vi "maxp.vi"() -> ()   [LabVIEW 2020]
uses:
  <vilib>/userdefined/High Color/IMAQdx.ctl
  C:/Users/lenovo/source/repos/MSMQ_try/how/bin/Release/how.dll
  source/repos/MSMQ_try/how/bin/Release/how.dll
  C:/Users/lenovo/source/repos/MSMQ_try/MIrror_x64/bin/Debug/MIrror_x64.dll
  source/repos/MSMQ_try/MIrror_x64/bin/Debug/MIrror_x64.dll
  <vilib>/vision/driver/NI_Vision_Acquisition_Software.lvlib
  source/repos/cont2019/x64/Release/Image_processing.dll
  <resource>/objmgr/imaqdx.rc
panel:
  in  "treshold":dbl=20000000.0
  out "st":bool
  out "ind":i32
  in  "ENA":bool
  in  "Relax":bool
  out "Power 2":dbl(graph)
  out "Power_val":dbl
  in  "stop 2":bool
  out "Image":T1(plugin-control)
  in  "Exposure time":dbl=1000.0
  out "FPS":dbl
  out "maximum":u8
  out "Power":dbl(graph)
  in  "Num frames":i32=3
  in  "Session In":T2="cam2"
  in  "amplitude_limit":dbl=0.1
  in  "phi_v":dbl
  in  "phi_g":dbl=1.6
  in  "phi_p":dbl=1.2
  in  "vel_limit":dbl=0.4
  in  "init_zero":bool
  out "Waveform Graph 2":dbl[](graph)
  in  "stop":bool
  out "mirror params":string
  in  "DM":bool
  out "Iterations":i32
  out "global_best_value":dbl
  out "Waveform Graph":dbl[](graph)
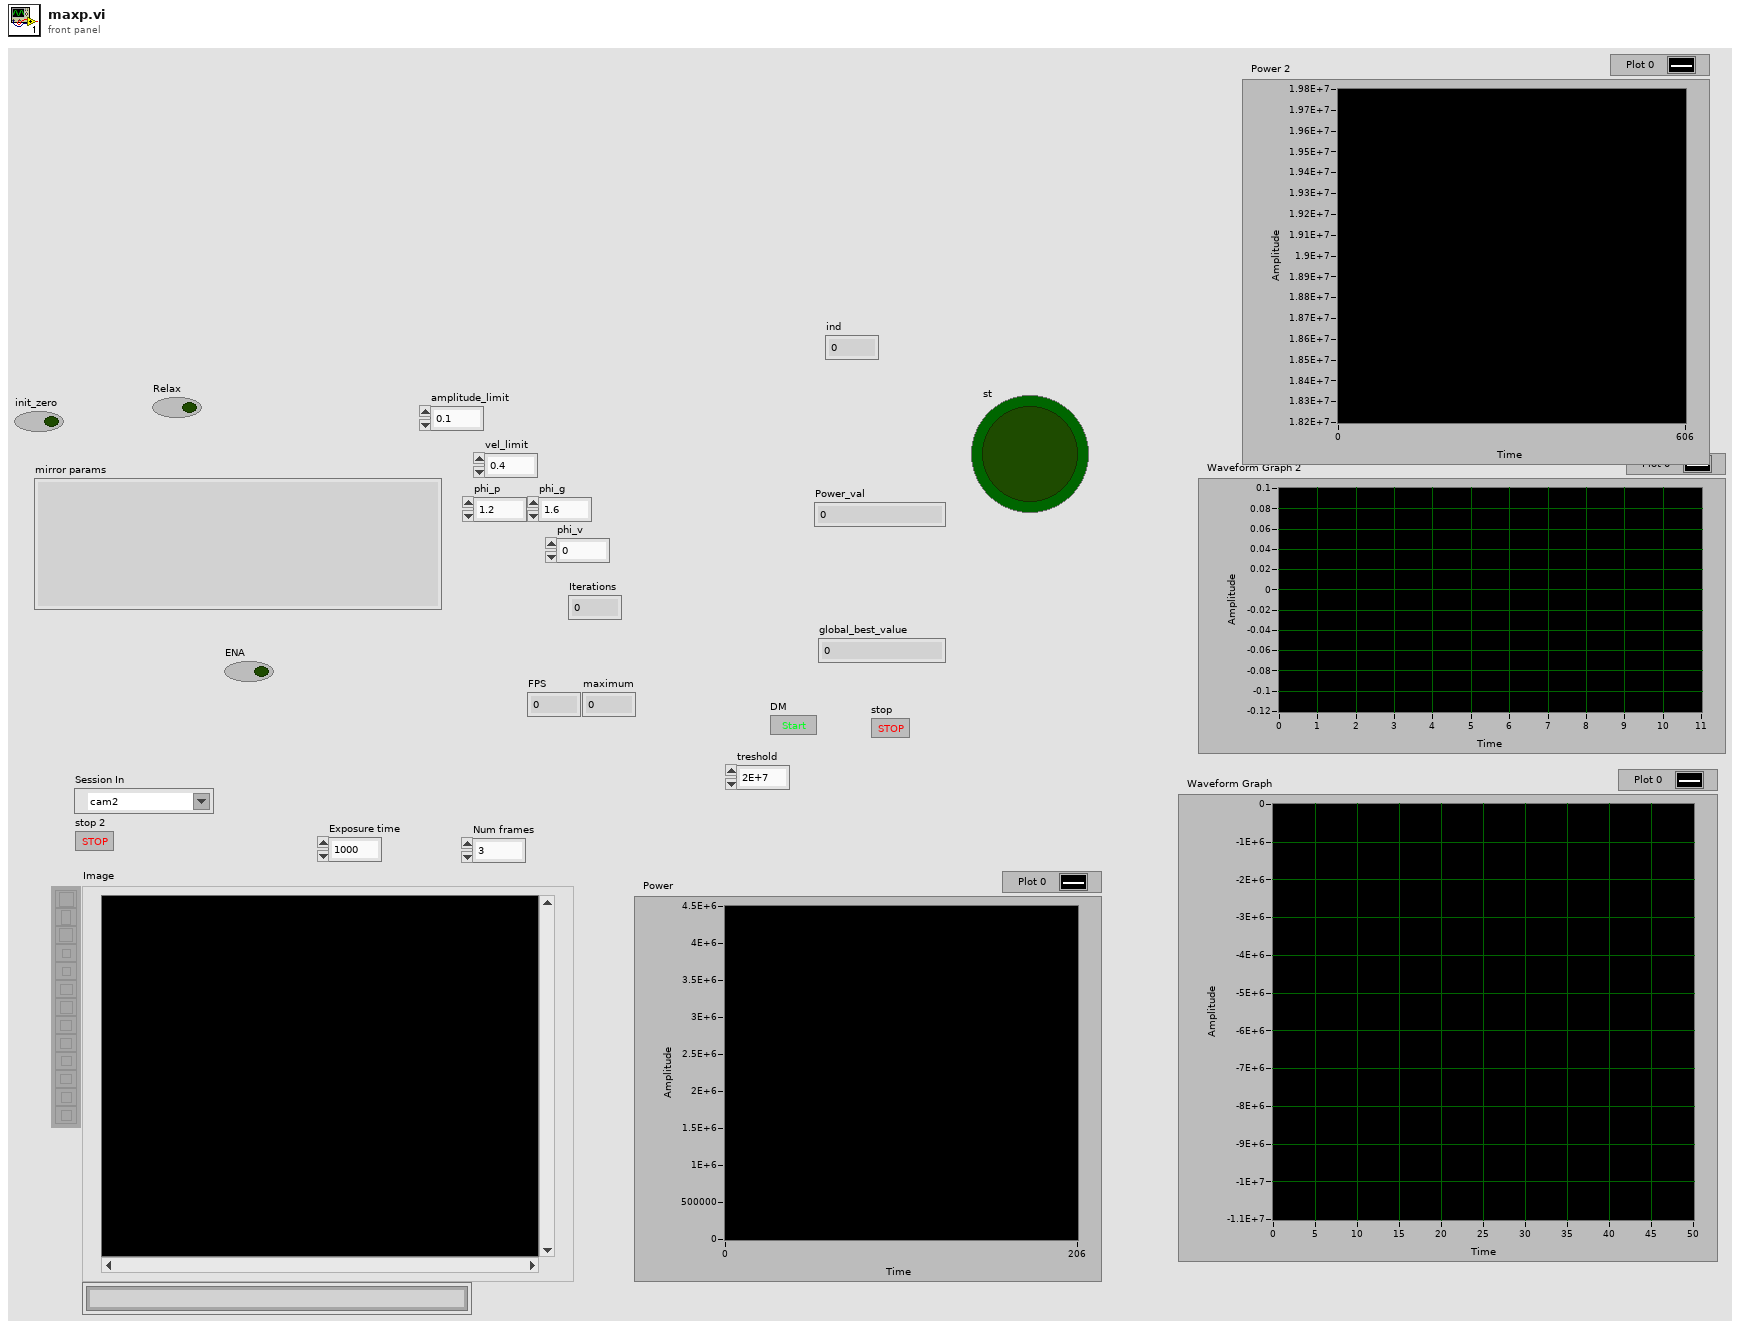
[diagram p1: front panel]
types:
  T1 = typedef "IMAQ Image.ctl" = refnum<image>
  T2 = typedef "IMAQdx.ctl" = refnum<k21>
  T3 = cluster{"Global Rectangle":i32[], "Contours":cluster{"Contour Type":u32, "ROI Type":u32, "Points":i32[]}[]}
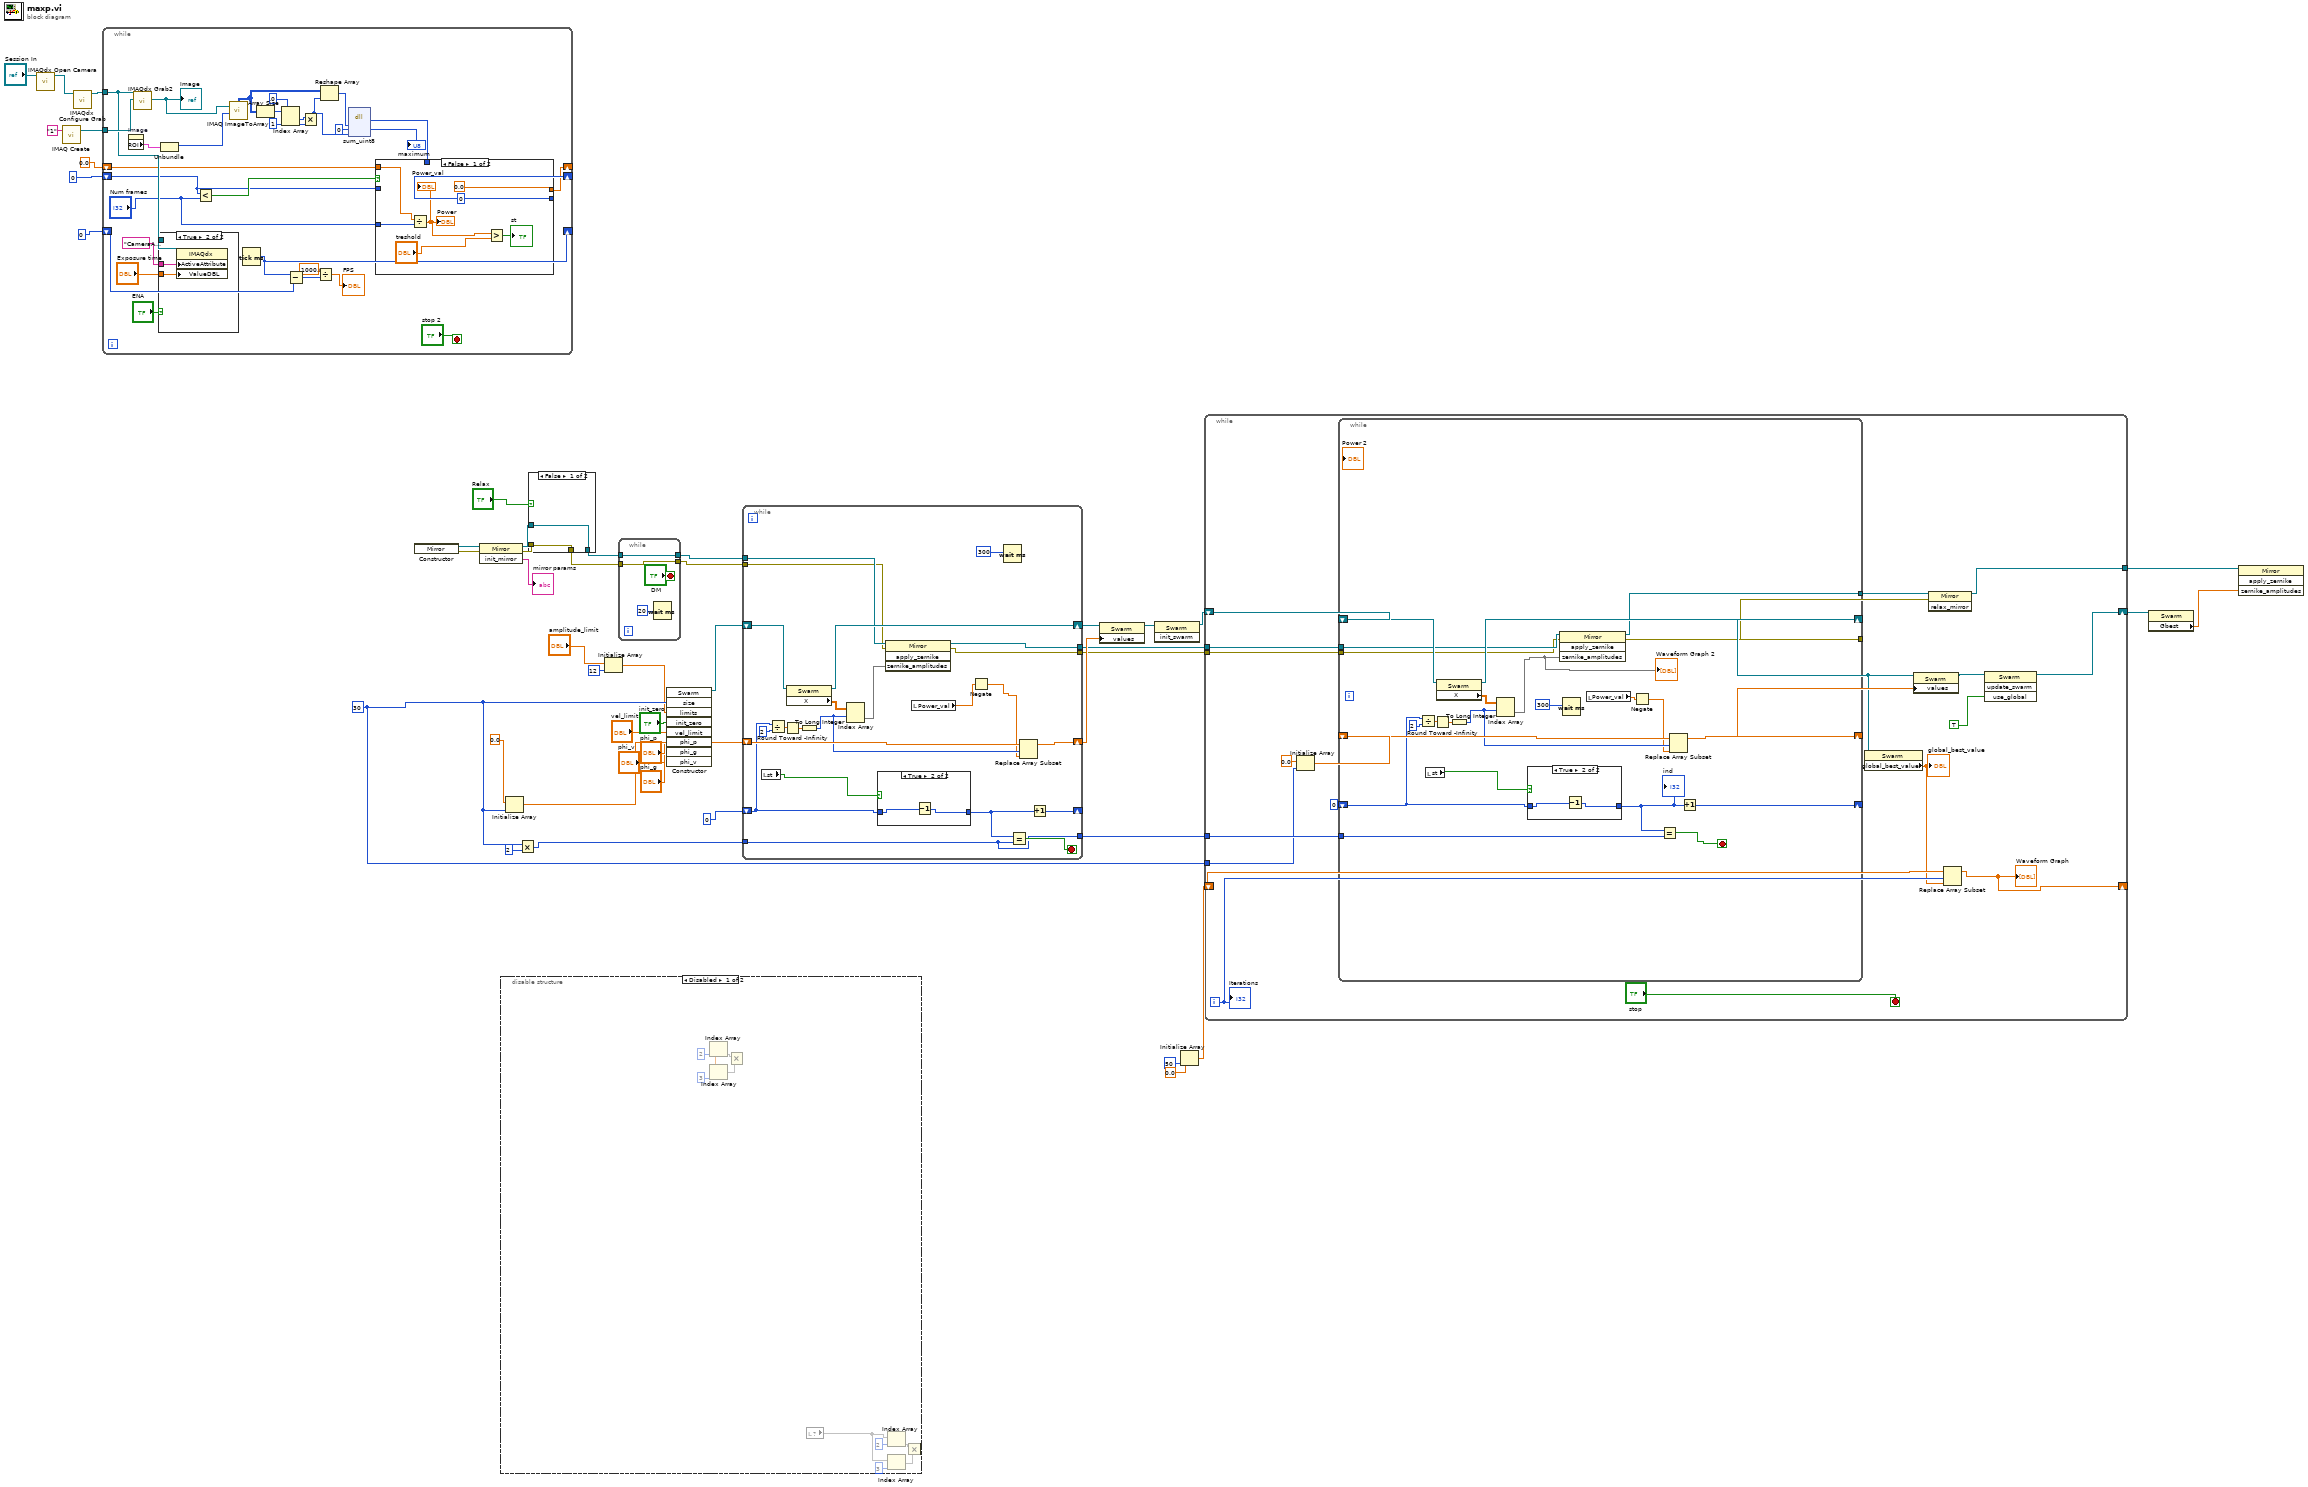
[diagram p0: block diagram]
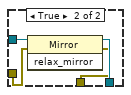
[diagram p2: hidden frame]
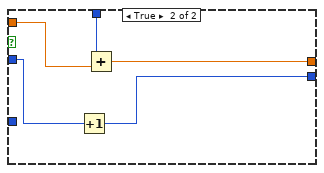
[diagram p7: hidden frame]
diagram:
  w27 = 30 ("size")
  n1 = call <vilib>:"IMAQdx Open Camera.vi"("Session In"="Session In") -> ("Session Out"=w45:T2)  [unwired: 9 in, 1 out]
  n2 = call "IMAQ Create"("Image Name"="1") -> ("New Image"=w42:T1)  [unwired: 4 in, 1 out]
  n3 = call <vilib>:"IMAQdx Configure Grab.vi"("Session In"=w45) -> ("Session Out"=w44:T2)  [unwired: 9 in, 1 out]
  n4 = while {
    tunnel: w44 -> [w59]
    tunnel: w42 -> [w66]
    shift-right: [w64] -> _
    shift-left: 0 -> [w65]
    shift-right: [w53] -> _
    shift-left: 0 -> [w54]
    shift-right: [w49] -> _
    shift-left: 0.0 -> [w51]
    stop <- "stop 2" stop-if-true
    n5 = property on="Image" class="ImageControl"() -> ("ROI"=w75:T3)  [unwired: 2 in, 2 out]
    n6 = call <vilib>:"IMAQdx Grab2.vi"("Image In"=w66, "Session In"=w59) -> ("Image Out"=w76:T1)  [unwired: 6 in, 3 out]
    "Image" <- w76
    n7 = case shown="True" "ENA" {
      tunnel: "Exposure time" -> [_ w80]
      tunnel: w59 -> [_ w79]
      tunnel: "CameraAttributes::AcquisitionControl::ExposureTime" ("ValueString") -> [_ w78]
      frame False {
      }
      frame True {
        n8 = property class="IMAQdx"(reference=w79, "ActiveAttribute"=w78, "ValueDBL"=w80) -> ()  [unwired: 1 in, 2 out]
      }
    }
    n9 = Unbundle(w75) -> ("Global Rectangle"=w74:i32[])  [unwired: 1 out]
    n10 = Less?(x=w54, y="Num frames") -> (x < y?=w55:bool)
    n11 = call "IMAQ ImageToArray"("Optional Rectangle"=w74, "Image"=w76) -> ("Image Pixels (U8)"=w68:u8[][])  [unwired: 2 in, 4 out]
    n12 = Tick Count (ms)() -> (millisecond timer value=w64:u32)
    n13 = Array Size(array=w68) -> (size(s)=w73:i32[])
    n14 = Index Array(array=w73, index #1=0 ("index"), index #2=1 ("index")) -> (element #1=w70:i32, element #2=w69:i32)
    n15 = Subtract(x=w64, y=w65) -> (x-y=w61:u32)
    n16 = Multiply(x=w70, y=w69) -> (x*y=w67:i32)
    n17 = Divide(x=1000.0, y=w61) -> (x/y=→"FPS":dbl)
    n18 = Reshape Array(w68, w67) -> (w57:u8[])
    n19 = dll-call lib="C:/Users/lenovo/source/repos/cont2019/x64/Release/Image_processing.dll" fn="sum_uint8"("pixel_data"=w57, "maximum"=u8 0, "lenght"=w67) -> ("sum"=w50:u64, "maximum"=→"maximum":u8)  [unwired: 5 in, 2 out]
    n20 = case shown="False" w55 {
      tunnel: w54 -> [_ w92]
      tunnel: [0 w91] -> w53
      tunnel: w51 -> [w84 w90]
      tunnel: w50 -> [_ w89]
      tunnel: [0.0 w88] -> w49
      tunnel: "Num frames" -> [w85 _]
      frame False {
        n21 = Divide(x=w84, y=w85) -> (x/y=w82:dbl)
        "Power" <- w82
        "Power_val" <- w82
        n22 = Greater?(x=w82, y="treshold") -> (0:→"st":bool)
      }
      frame True {
        n23 = Increment(x=w92) -> (x+1=w91:i32)
        n24 = Add(x=w89, y=w90) -> (x+y=w88:dbl)
      }
    }
  }
  n25 = constructor class="Mirror"() -> (reference out=w23:refnum<k24>, error out=w21:errorcluster)  [unwired: 3 in, 1 out]
  n26 = invoke class="Mirror" method="init_mirror"(reference=w23, error in=w21) -> (reference out=w16:refnum<k24>, error out=w15:errorcluster, "init_mirror"=→"mirror params":string)  [unwired: 1 in]
  n27 = disable-structure shown="Disabled" {
    frame Disabled {
      n28 = Index Array(index=3) -> (array=w93:dbl[], element=w97)
      n29 = Index Array(array=w93, index=2) -> (element=w96)
      n30 = Multiply(x=w96, y=w97) -> ()  [unwired: 1 out]
      n31 = local read item#-1() -> (w98)
      n32 = Index Array(array=w98, index=2) -> (element=w101)
      n33 = Index Array(array=w98, index=3) -> (element=w102)
      n34 = Multiply(x=w101, y=w102) -> ()  [unwired: 1 out]
    }
    frame Enabled {
    }
  }
  n35 = Initialize Array(0.0 ("element"), w27) -> (w35:dbl[])
  n36 = Multiply(x=w27, y=2) -> (x*y=w30:i32)
  n37 = case shown="False" "Relax" {
    tunnel: w16 -> [w103 w108]
    tunnel: w15 -> [w104 w107]
    tunnel: [w103 w106] -> w14
    tunnel: [w104 w105] -> w13
    frame False {
    }
    frame True {
      n38 = invoke class="Mirror" method="relax_mirror"(reference=w108, error in=w107) -> (reference out=w106:refnum<k24>, error out=w105:errorcluster)  [unwired: 1 in, 1 out]
    }
  }
  n39 = Initialize Array("amplitude_limit", 12 ("dimension size")) -> (w5:dbl[])
  n40 = while {
    tunnel: [w111] -> w20
    tunnel: w14 -> [w111]
    tunnel: [w109] -> w19
    tunnel: w13 -> [w109]
    stop <- "DM" stop-if-true
    n41 = Wait (ms)(milliseconds to wait=u32 20) -> ()  [unwired: 1 out]
  }
  n42 = constructor class="Swarm"("size"=w27, "limits"=w5, "init_zero"="init_zero", "vel_limit"="vel_limit", "phi_p"="phi_p", "phi_g"="phi_g", "phi_v"="phi_v") -> (reference out=w36:refnum<k24>)  [unwired: 3 in, 9 out]
  n43 = while {
    shift-right: [w128] -> w33
    shift-left: w35 -> [w129]
    shift-right: [w126] -> w34
    shift-left: w36 -> [w135]
    shift-right: [w125] -> _
    shift-left: 0 -> [w123]
    tunnel: w30 -> [w121]
    tunnel: [w121] -> w28
    tunnel: w20 -> [w120]
    tunnel: w19 -> [w118]
    tunnel: [w117] -> w18
    tunnel: [w116] -> w17
    stop <- w124 stop-if-true
    n44 = local read "st"() -> (w113:bool)
    n45 = Divide(x=w123, y=2) -> (x/y=w133:dbl)
    n46 = Round Toward -Infinity(1:w133) -> (0:w132:dbl)
    n47 = property class="Swarm"(reference=w135) -> (reference out=w126:refnum<k24>, "X"=w131:dbl[][])  [unwired: 1 in, 1 out]
    n48 = To Long Integer(number=w132) -> (32bit integer=w127:i32)
    n49 = Index Array(array=w131, index (row)=w127) -> (element=w119:dbl[])  [unwired: 1 in]
    n50 = case shown="True" w113 {
      tunnel: w123 -> [w136 w138]
      tunnel: [w136 w137] -> w122
      frame False {
      }
      frame True {
        n51 = Decrement(x=w138) -> (x-1=w137:i32)
      }
    }
    n52 = invoke class="Mirror" method="apply_zernike"(reference=w120, error in=w118, "zernike_amplitudes"=w119) -> (reference out=w117:refnum<k24>, error out=w116:errorcluster)  [unwired: 1 in, 2 out]
    n53 = local read "Power_val"() -> (w114:dbl)
    n54 = Negate(x=w114) -> (-x=w115:dbl)
    n55 = Wait (ms)(milliseconds to wait=u32 300) -> ()  [unwired: 1 out]
    n56 = Equal?(x=w122, y=w121) -> (x = y?=w124:bool)
    n57 = Replace Array Subset(array=w129, new element=w115, index=w127) -> (w128:dbl[])
    n58 = Increment(x=w122) -> (x+1=w125:i32)
  }
  n59 = property class="Swarm"(reference=w34, "values"=w33) -> (reference out=w32:refnum<k24>)  [unwired: 1 in, 1 out]
  n60 = invoke class="Swarm" method="init_swarm"(reference=w32) -> (reference out=w29:refnum<k24>)  [unwired: 2 in, 2 out]
  n61 = Initialize Array(0.0 ("element"), 50 ("dimension size")) -> (w24:dbl[])
  n62 = while {
    tunnel: w28 -> [w157]
    tunnel: w27 -> [w156]
    shift-right: [w150] -> w3
    shift-left: w29 -> [w159]
    shift-right: [w145] -> _
    shift-left: w24 -> [w148]
    tunnel: w18 -> [w144]
    tunnel: w17 -> [w143]
    tunnel: [w139] -> w4
    i -> [w147]
    stop <- "stop" stop-if-true
    n63 = Initialize Array(0.0 ("element"), w156) -> (w154:dbl[])
    n64 = while {
      shift-right: [w175] -> w153
      shift-left: w154 -> [w176]
      shift-right: [w173] -> w149
      shift-left: w159 -> [w182]
      shift-right: [w172] -> _
      shift-left: 0 -> [w170]
      tunnel: w157 -> [w171]
      tunnel: w144 -> [w168]
      tunnel: w143 -> [w167]
      tunnel: [w166] -> w142
      tunnel: [w165] -> w141
      stop <- w164 stop-if-true
      n65 = Divide(x=w170, y=2) -> (x/y=w180:dbl)
      n66 = local read "st"() -> (w160:bool)
      n67 = Round Toward -Infinity(1:w180) -> (0:w179:dbl)
      n68 = property class="Swarm"(reference=w182) -> (reference out=w173:refnum<k24>, "X"=w178:dbl[][])  [unwired: 1 in, 1 out]
      n69 = To Long Integer(number=w179) -> (32bit integer=w174:i32)
      n70 = Index Array(array=w178, index (row)=w174) -> (element=w163:dbl[])  [unwired: 1 in]
      "Waveform Graph 2" <- w163
      n71 = case shown="True" w160 {
        tunnel: w170 -> [w183 w185]
        tunnel: [w183 w184] -> w169
        frame False {
        }
        frame True {
          n72 = Decrement(x=w185) -> (x-1=w184:i32)
        }
      }
      "ind" <- w169
      n73 = invoke class="Mirror" method="apply_zernike"(reference=w168, error in=w167, "zernike_amplitudes"=w163) -> (reference out=w166:refnum<k24>, error out=w165:errorcluster)  [unwired: 1 in, 2 out]
      n74 = Wait (ms)(milliseconds to wait=u32 300) -> ()  [unwired: 1 out]
      n75 = local read "Power_val"() -> (w161:dbl)
      n76 = Negate(x=w161) -> (-x=w162:dbl)
      n77 = Equal?(x=w169, y=w171) -> (x = y?=w164:bool)
      n78 = Replace Array Subset(array=w176, new element=w162, index=w174) -> (w175:dbl[])
      n79 = Increment(x=w169) -> (x+1=w172:i32)
    }
    n80 = property class="Swarm"(reference=w149) -> ("global_best_value"=w146:dbl)  [unwired: 1 in, 2 out]
    "global_best_value" <- w146
    n81 = property class="Swarm"(reference=w149, "values"=w153) -> (reference out=w152:refnum<k24>)  [unwired: 1 in, 1 out]
    n82 = invoke class="Mirror" method="relax_mirror"(reference=w142, error in=w141) -> (reference out=w139:refnum<k24>)  [unwired: 1 in, 2 out]
    n83 = Replace Array Subset(array=w148, new element=w146, index=w147) -> (w145:dbl[])
    "Waveform Graph" <- w145
    n84 = invoke class="Swarm" method="update_swarm"(reference=w152, "use_global"=TRUE) -> (reference out=w150:refnum<k24>)  [unwired: 2 in, 3 out]
    "Iterations" <- w147
  }
  n85 = property class="Swarm"(reference=w3) -> ("Gbest"=w2:dbl[])  [unwired: 1 in, 2 out]
  n86 = invoke class="Mirror" method="apply_zernike"(reference=w4, "zernike_amplitudes"=w2) -> ()  [unwired: 2 in, 4 out]
